vi "Untitled 1.vi"() -> ()   [LabVIEW 2017]
panel:
  out "return code":i32
  out "error out":errorcluster
  out "standard output":string
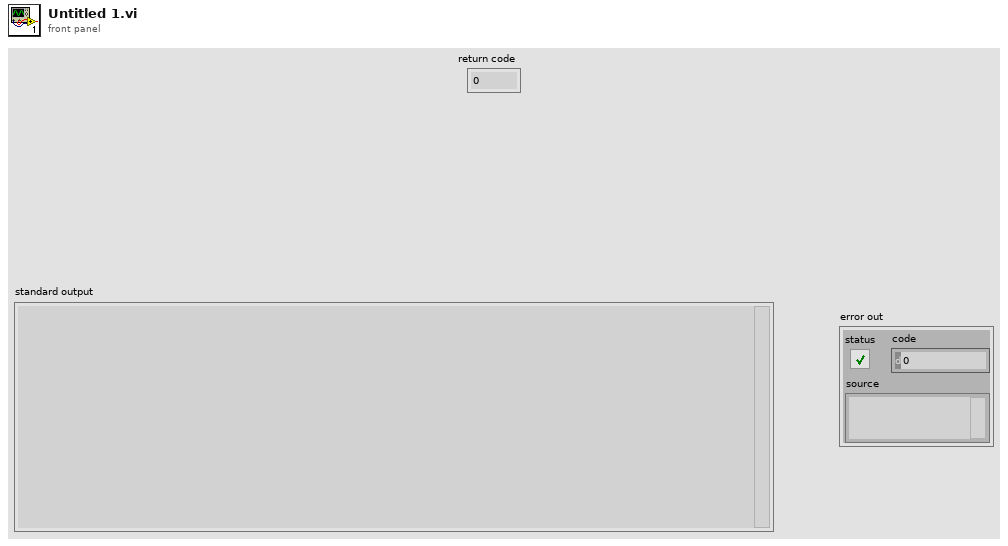
[diagram p1: front panel]
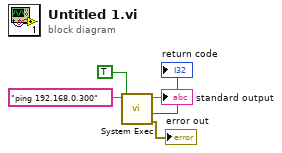
[diagram p0: block diagram]
diagram:
  n1 = call <vilib>:"System Exec.vi"("wait until completion? (T)"=TRUE, "command line"="ping 192.168.0.300") -> ("error out"=→"error out":errorcluster, "return code"=→"return code":i32, "standard output"=→"standard output":string)  [unwired: 6 in, 1 out]
